vi "Step2_Touch.vi"   [LabVIEW 2012]
uses:
  <vilib>/NXT/Subs/MotorOutput.ctl
  <vilib>/NXT/Block Support/NXT_InputPort.ctl
types:
  T1 = typedef "NXT_InputPort.ctl" = u32
  T2 = typedef "MotorOutput.ctl" = u8
  T3 = typedef "LVHSConnector.ctl" = refnum<class "BrickReference.lvclass">
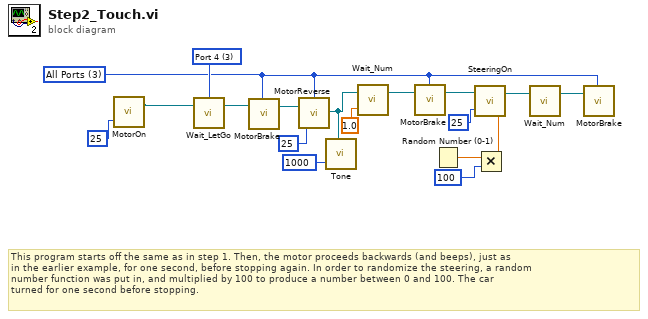
[diagram p0: block diagram]
diagram:
  w18 = T1 3 items=["Port 1", "Port 2", "Port 3", "Port 4"] ("Port (Port 1)")
  w1 = T2 3 items=["Port A"=0, "Port B"=1, "Port C"=2, "Ports A & B"=4, "Ports A & C"=5, "Ports B & C"=6, "All Ports"=3] ("Output Port (All Ports)")
  # "This program starts off the same as in step 1. Then, the motor proceeds backwards (and beeps), just as\nin the earlier example, for one second, before stopping again. In order to randomize the steering, a random\nnumber function was put in, and multiplied by 100 to produce a number between 0 and 100. The car \nturned for one second before stopping."
  n1 = call <vilib>:"MotorOn.vi"("Power (75)"=25) -> ("NXT/EV3"=w10:T3)  [unwired: 3 in]
  n2 = call <vilib>:"Wait_LetGo.vi"("NXT/EV3"=w10, "Port (Port 1)"=w18) -> ("NXTEV3"=w17:T3)  [unwired: 2 in]
  n3 = call <vilib>:"MotorBrake.vi"("NXT/EV3"=w17, "Port (All Ports)"=w1) -> ("NXT/EV3"=w16:T3)  [unwired: 2 in]
  n4 = call <vilib>:"MotorReverse.vi"("Power (75)"=25, "NXT/EV3"=w16, "Output Port (All Ports)"=w1) -> ("NXT/EV3"=w15:T3)  [unwired: 1 in]
  n5 = call <vilib>:"Tone.vi"("Duration (500 ms)"=u16 1000, "NXT/EV3"=w15) -> ()  [unwired: 2 in, 1 out]
  n6 = call <vilib>:"Wait_Num.vi"("Time (1 sec)"=sgl 1.0, "NXT/EV3"=w15) -> ("NXT/EV3"=w14:T3)  [unwired: 2 in]
  n7 = call <vilib>:"MotorBrake.vi"("NXT/EV3"=w14, "Port (All Ports)"=w1) -> ("NXT/EV3"=w13:T3)  [unwired: 2 in]
  n8 = Random Number (0-1)() -> (number: 0 to 1=w8:dbl)
  n9 = Multiply(x=w8, y=100) -> (x*y=w6:dbl)
  n10 = call <vilib>:"SteeringOn.vi"("Power (75)"=25, "Steering (100)"=w6, "NXT/EV3"=w13) -> ("NXT/EV3"=w3:T3)  [unwired: 1 in]
  n11 = call <vilib>:"Wait_Num.vi"("NXT/EV3"=w3) -> ("NXT/EV3"=w2:T3)  [unwired: 3 in]
  n12 = call <vilib>:"MotorBrake.vi"("NXT/EV3"=w2, "Port (All Ports)"=w1) -> ()  [unwired: 2 in, 1 out]
